vi "PH_AWG-510.Close.vi"(0 "VI in":refnum<vi>, 5 "error in (no error)":errorcluster) -> (14 "VI out":refnum<vi>, 19 "error out":errorcluster)   [LabVIEW 2014, in "PH_AWG-510.lvlib"]
doc: "This VI closes the VISA session and sets related own attributes."
uses:
  PH_AWG-510.lvlib
  instr.lib/awg510/Tektronix AWG510 - Driver.lvlib
  PH_Common/PH_Common.lvlib
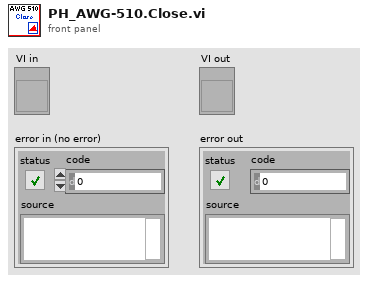
[diagram p1: front panel]
types:
  T1 = typedef "PH_AWG-510.lvlib/PH_AWG-510.i attribute.ctl" = cluster{"GUI Refs":cluster{"Delete":refnum<vi>, "Trigger Settings":refnum<vi>, "Start Device":refnum<vi>, "Instrument Information":refnum<vi>, "Lock Frontpanel":refnum<vi>, "Waveform Pattern File":refnum<vi>, "Initialize":refnum<vi>, "Output Settings":refnum<vi>}, "Instrument Information":T2, "Initialized?":bool, "Current Settings":cluster{"Trigger":T3, "Output Settings":T4}, "Wanted Settings":cluster{"Trigger":T3, "Output Settings":T4}, "Device frontpanel locked?":bool, "Default File Path":path}
  T2 = typedef "PH_AWG-510.lvlib/PH_AWG-510.Instrument Information Dataset.ctl" = cluster{"VISA resource name":refnum<visa-resource-name>, "Instrument Firmware Revision":string, "Manufacturer":string, "Model":string, "Serial Number":string, "Error Message":string, "Device Status":enum16{"stopped", "wating for trigger", "running", "Failure"}}
  T3 = typedef "PH_AWG-510.lvlib/PH_AWG-510.Trigger Settings.ctl" = cluster{"Mode":enum16{"Continuous", "Triggered", "Gated", "Enhanced"}, "Level (V)":dbl, "External Source":bool}
  T4 = typedef "PH_AWG-510.lvlib/PH_AWG-510.Output Settings.ctl" = cluster{"Activate Channel":bool, "VPP (V)":dbl, "Clock (Hz)":dbl, "File Name (Device)":string, "#1":u16, "#2":u16, "#3":u16, "#4":u16, "#5":u16, "#6":u16, "#7":u16, "#8":u16, "#9":u16, "#10":u16, "#11":u16, "#12":u16, "#13":u16, "#14":u16, "#15":u16, "#16":u16, "#17":u16, "#18":u16, "#19":u16, "#20":u16, "Offset (V)":dbl}
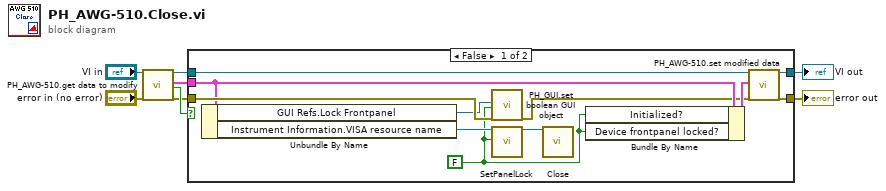
[diagram p0: block diagram]
diagram:
  n1 = call "PH_AWG-510.get data to modify.vi"("i ref in"="VI in", "error in (no error)"="error in (no error)") -> ("i ref out"=w5:refnum<vi>, "i attribute"=w7:T1, "timed out"=w8:bool, "error out"=w2:errorcluster)  [unwired: 14 in]
  n2 = case shown="False" w8 {
    tunnel: w2 -> [w19 w20]
    tunnel: [w18 w20] -> w3
    tunnel: w5 -> [w17 w21]
    tunnel: [w16 w21] -> w6
    tunnel: w7 -> [w14 _]
    frame False {
      w9 = FALSE ("Status (Lock)")
      n3 = Unbundle By Name(w14) -> ("GUI Refs.Lock Frontpanel"=w10:refnum<vi>, "Instrument Information.VISA resource name"=w13:refnum<visa-resource-name>)
      n4 = call "PH_GUI.set boolean GUI object.vi"("Boolean Knob GUI Ref"=w10, "Value"=w9, "error in (no error)"=w19) -> ("error out"=w11:errorcluster)  [unwired: 16 in]
      n5 = call "SetPanelLock.vi"("VISA resource name"=w13, "Status (Lock)"=w9) -> ("VISA resource name out"=w12:refnum<visa-resource-name>)  [unwired: 16 in, 1 out]
      n6 = call "Close.vi"("VISA resource name"=w12) -> ()  [unwired: 18 in, 1 out]
      n7 = Bundle By Name(cluster=w14, "Initialized?"=w9, "Device frontpanel locked?"=w9) -> (w15:T1)
      n8 = call "PH_AWG-510.set modified data.vi"("i ref in"=w17, "i attribute"=w15, "error in (no error)"=w11) -> ("i ref out"=w16:refnum<vi>, "error out"=w18:errorcluster)  [unwired: 15 in]
    }
    frame True {
    }
  }
  "VI out" <- w6
  "error out" <- w3
